vi "Close_Instr.vi"(8 "error in (no error)":errorcluster caption="entrée d'erreur (pas d'erreur)", 11 "Class DIO en entrée":refnum<class "Class Instrument Log_File.lvclass">) -> (0 "error out":errorcluster caption="sortie d'erreur", 3 "Class DIO en Sortie":refnum<class "Class Instrument Log_File.lvclass">)   [LabVIEW 2020, in "Library Instrument & Equipement.lvlib" / "Library Instruments.lvlib" / "Class Instrument Log_File.lvclass"]
uses:
  Class Instrument Log_File.lvclass
  Class Instrument Log_File.lvclass/Class Instrument Log_File.ctl
  Log File/Class Log_File Altyor/Class Log_File Altyor.lvclass
  Instrument (Default)/Class Instrument (Default).lvclass
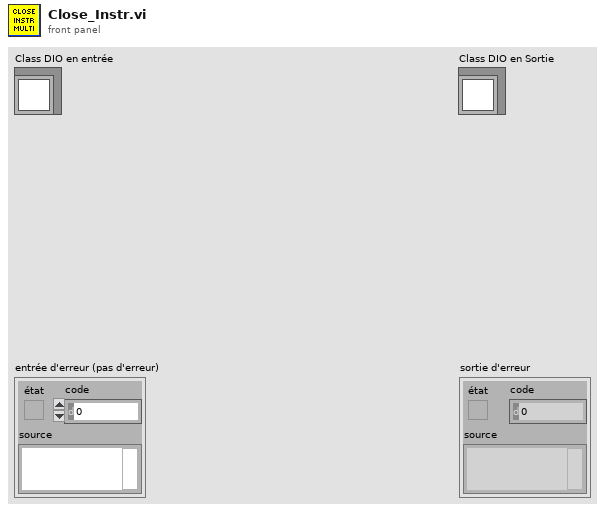
[diagram p1: front panel]
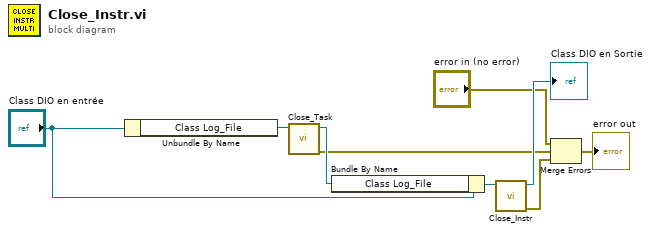
[diagram p0: block diagram]
diagram:
  n1 = Unbundle By Name("Class DIO en entrée") -> ("Class Log_File"=w3:refnum<class "Class Log_File Altyor.lvclass">)
  n2 = call-dynamic "Close_Task.vi"("Class Log_File Altyor en entrée"=w3) -> ("error out"=w1:errorcluster, "Class Log_File Altyor en sortie"=w2:refnum<class "Class Log_File Altyor.lvclass">)  [unwired: 9 in]
  n3 = Bundle By Name(cluster="Class DIO en entrée", "Class Log_File"=w2) -> (w7:refnum<class "Class Instrument Log_File.lvclass">)
  n4 = call-parent "Close_Instr.vi"("Class Instrument (Default) en entrée"=w7) -> ("error out"=w5:errorcluster, "Class Instrument (Default) en sortie"=→"Class DIO en Sortie":refnum<class "Class Instrument Log_File.lvclass">)  [unwired: 9 in]
  n5 = Merge Errors("error in (no error)", w1, w5) -> (→"error out":errorcluster)
